vi "Traffic lights.vi"() -> ()   [LabVIEW 2012]
doc: "Use this template to build a standard state machine design pattern. Each state executes code and determines which state to transition to. Contrast this design pattern with the User Interface Event Handler pattern, in which code executes in response to user actions. Contrast this design pattern also with the Queued Message Handler pattern, in which each message handling code can queue zero or more new messages.\nNote: This template does not contain the most recent programming guidelines recommended by National Instruments. For a complete, project-based implementation of the Standard State Machine pattern, use the Create Project dialog box instead of this template."
uses:
  swiatla.ctl
  <vilib>/DAQmx/write.llb/DAQmx Write (Digital 1D Bool 1Chan 1Samp).vi
  <vilib>/DAQmx/create/channels.llb/DAQmx Create Channel (DO-Digital Output).vi
  <vilib>/DAQmx/miscellaneous.llb/DAQmx Fill In Error Info.vi
panel:
  in  "Numeric":dbl=20.0
  in  "pomaranczowe":bool
  in  "stop":bool
  in  "DAQmx Physical Channel":tag="Dev4/port0/line0:5"
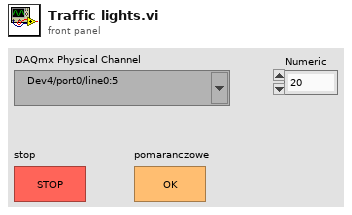
[diagram p1: front panel]
types:
  T1 = typedef "swiatla.ctl" = enum16{"Initialize", "Czerwone", "Czerwono-pomaranczowe", "Zielone", "Pomaranczowe", "Migajace_pomarancz", "Podw_czerw", "Powd_czerw_pomaran", "Mig_zgasz", "Stop"}
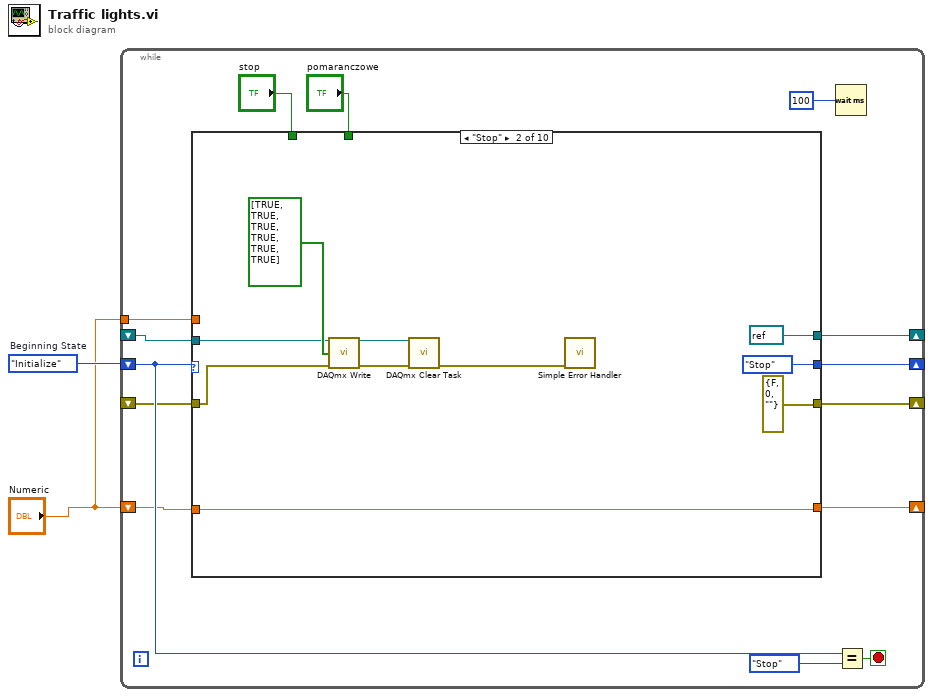
[diagram p0: block diagram]
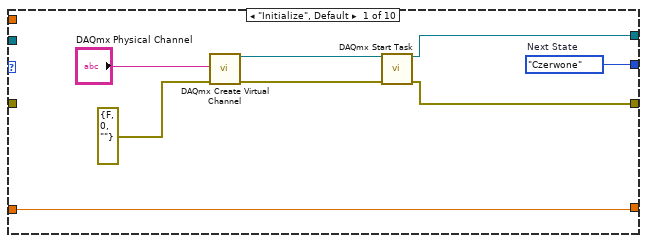
[diagram p2: hidden frame]
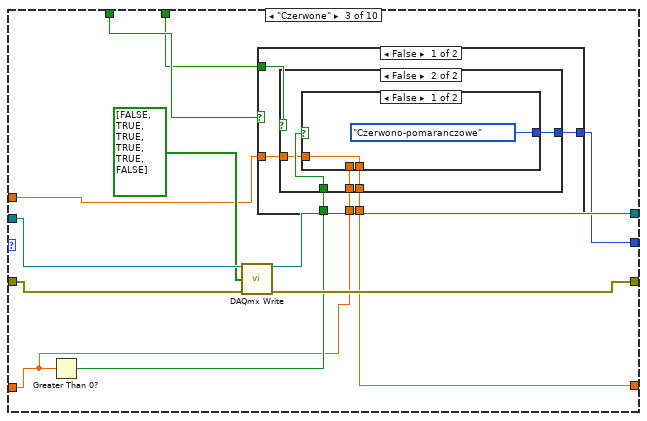
[diagram p3: hidden frame]
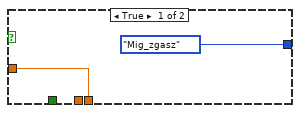
[diagram p4: hidden frame]
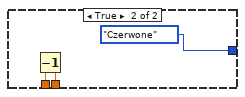
[diagram p5: hidden frame]
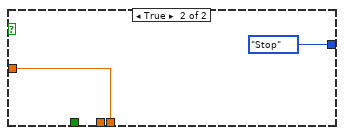
[diagram p6: hidden frame]
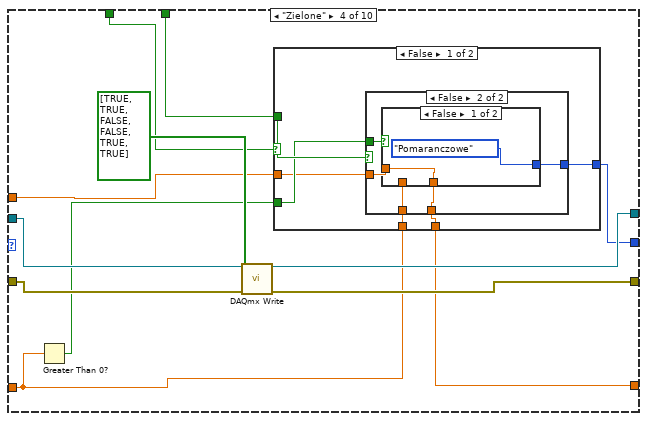
[diagram p7: hidden frame]
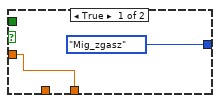
[diagram p8: hidden frame]
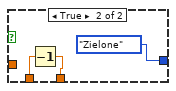
[diagram p9: hidden frame]
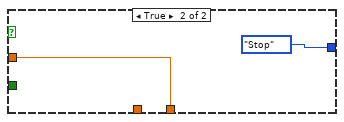
[diagram p10: hidden frame]
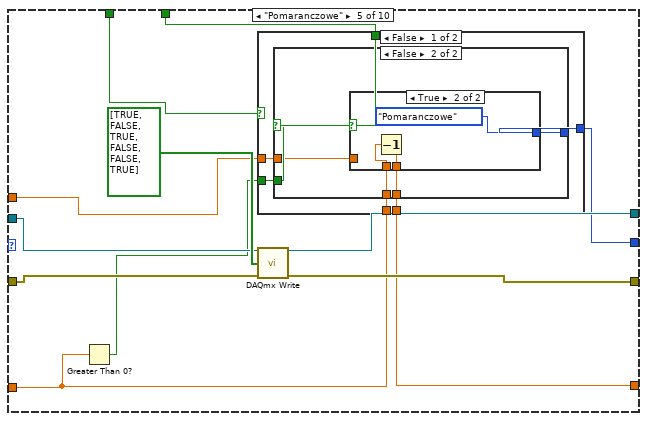
[diagram p11: hidden frame]
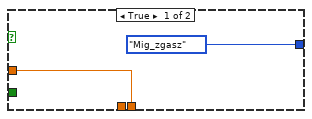
[diagram p12: hidden frame]
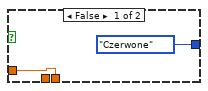
[diagram p13: hidden frame]
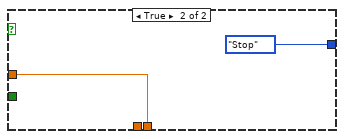
[diagram p14: hidden frame]
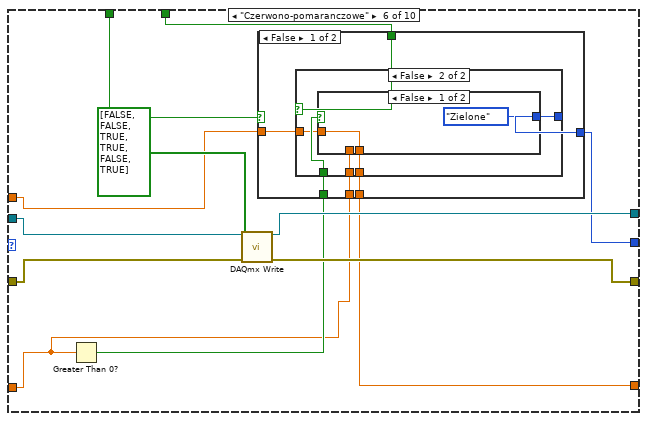
[diagram p15: hidden frame]
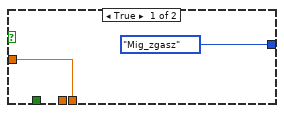
[diagram p16: hidden frame]
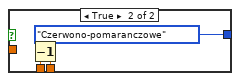
[diagram p17: hidden frame]
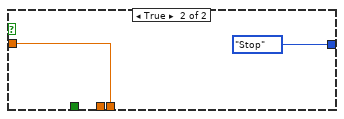
[diagram p18: hidden frame]
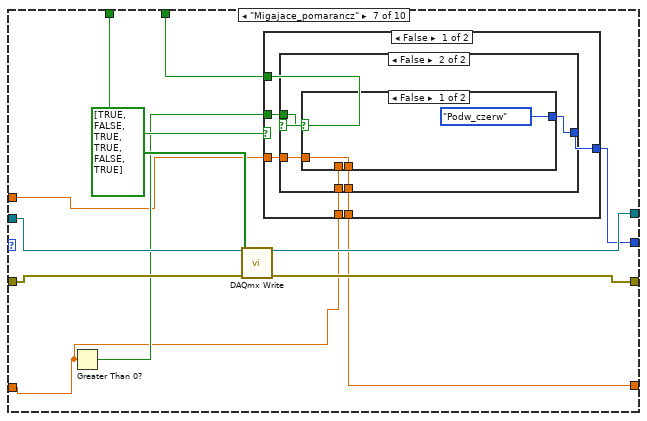
[diagram p19: hidden frame]
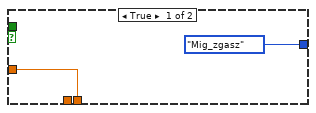
[diagram p20: hidden frame]
diagram:
  w2 = swiatla."Initialize"  # Beginning State
  n1 = while {
    shift-right: [w13] -> _
    shift-left: w2 -> [w14]
    shift-right: [w10] -> _
    shift-left: _ -> [w8]
    shift-right: [w11] -> _
    shift-left: _ -> [w9]
    shift-right: [w4] -> _
    shift-left: "Numeric" -> [w5]
    tunnel: "Numeric" -> [w3]
    stop <- w16 stop-if-true
    n2 = case shown="\"Stop\"" w14 {
      tunnel: [w24 swiatla."Stop" ("Next State") w40 w72 w104 w136 w168 w200 w232 w264] -> w13
      tunnel: [w20 refnum<k21> refnum ("task out") w43 w74 w109 w138 w170 w202 w234 w266] -> w11
      tunnel: [w19 errorcluster {"status"=FALSE, "code"=0, "source"=""} ("error out") w42 w75 w108 w139 w169 w201 w233 w265] -> w10
      tunnel: w9 -> [_ w29 w46 w77 w107 w141 w172 w204 w236 w268]
      tunnel: w8 -> [_ w28 w45 w76 w106 w140 w171 w203 w235 w267]
      tunnel: "stop" -> [_ _ w41 w73 w105 w137 w173 w205 w237 w269]
      tunnel: "pomaranczowe" -> [_ _ w39 w71 w103 w135 w167 w199 w231 w263]
      tunnel: w5 -> [w17 w25 w37 w69 w101 w133 w165 w197 w229 w261]
      tunnel: [w17 w25 w36 w68 w100 w132 w164 w196 w228 w260] -> w4
      tunnel: w3 -> [_ _ w35 w67 w99 w131 w163 w195 w227 w259]
      frame "Initialize", Default {
        w24 = swiatla."Czerwone"  # Next State
        n3 = call-poly <vilib>:"DAQmx Create Virtual Channel.vi"("lines"="DAQmx Physical Channel", "error in"=errorcluster {"status"=FALSE, "code"=0, "source"=""}) -> ("task out"=w22:refnum<k21>, "error out"=w21:errorcluster)  [unwired: 12 in]
        n4 = call <vilib>:"DAQmx Start Task.vi"("task/channels in"=w22, "error in"=w21) -> ("task out"=w20:refnum<k21>, "error out"=w19:errorcluster)  [unwired: 12 in]
      }
      frame "Stop" {
        n5 = call-poly <vilib>:"DAQmx Write.vi"("task/channels in"=w29, "data"=bool[] [TRUE, TRUE, TRUE, TRUE, TRUE, TRUE], "error in"=w28) -> ("task out"=w31:refnum<k21>, "error out"=w30:errorcluster)  [unwired: 10 in, 1 out]
        n6 = call <vilib>:"DAQmx Clear Task.vi"("task in"=w31, "error in"=w30) -> ("error out"=w33:errorcluster)  [unwired: 13 in]
        n7 = call <vilib>:"Simple Error Handler.vi"("error in (no error)"=w33) -> ()  [unwired: 4 in, 5 out]
      }
      frame "Czerwone" {
        n8 = Greater Than 0?(x=w37) -> (x > 0?=w38:bool)
        n9 = call-poly <vilib>:"DAQmx Write.vi"("task/channels in"=w46, "data"=bool[] [FALSE, TRUE, TRUE, TRUE, TRUE, FALSE], "error in"=w45) -> ("task out"=w43:refnum<k21>, "error out"=w42:errorcluster)  [unwired: 10 in, 1 out]
        n10 = case shown="False" w41 {
          tunnel: [w52 swiatla."Stop" ("Next State")] -> w40
          tunnel: w39 -> [w51 _]
          tunnel: w38 -> [w50 _]
          tunnel: w37 -> [w49 _]
          tunnel: [w48 w65] -> w36
          tunnel: w35 -> [w47 w65]
          frame False {
            n11 = case shown="False" w51 {
              tunnel: [swiatla."Mig_zgasz" ("Next State") w59] -> w52
              tunnel: w50 -> [_ w58]
              tunnel: w49 -> [_ w57]
              tunnel: [w53 w56] -> w48
              tunnel: w47 -> [w53 w55]
              frame True {
              }
              frame False {
                n12 = case shown="False" w58 {
                  tunnel: [swiatla."Czerwono-pomaranczowe" ("Next State") swiatla."Czerwone" ("Next State")] -> w59
                  tunnel: w57 -> [_ w63]
                  tunnel: [w60 w62] -> w56
                  tunnel: w55 -> [w60 _]
                  frame False {
                  }
                  frame True {
                    n13 = Decrement(x=w63) -> (x-1=w62:dbl)
                  }
                }
              }
            }
          }
          frame True {
          }
        }
      }
      frame "Zielone" {
        n14 = Greater Than 0?(x=w69) -> (x > 0?=w70:bool)
        n15 = call-poly <vilib>:"DAQmx Write.vi"("task/channels in"=w77, "data"=bool[] [TRUE, TRUE, FALSE, FALSE, TRUE, TRUE], "error in"=w76) -> ("task out"=w74:refnum<k21>, "error out"=w75:errorcluster)  [unwired: 10 in, 1 out]
        n16 = case shown="False" w73 {
          tunnel: [w84 swiatla."Stop" ("Next State")] -> w72
          tunnel: w71 -> [w83 _]
          tunnel: w70 -> [w82 _]
          tunnel: w69 -> [w81 _]
          tunnel: [w80 w97] -> w68
          tunnel: w67 -> [w79 w97]
          frame False {
            n17 = case shown="False" w83 {
              tunnel: [swiatla."Mig_zgasz" ("Next State") w91] -> w84
              tunnel: w82 -> [_ w90]
              tunnel: w81 -> [_ w89]
              tunnel: [w85 w88] -> w80
              tunnel: w79 -> [w85 w87]
              frame True {
              }
              frame False {
                n18 = case shown="False" w90 {
                  tunnel: [swiatla."Pomaranczowe" ("Next State") swiatla."Zielone" ("Next State")] -> w91
                  tunnel: w89 -> [_ w95]
                  tunnel: [w92 w94] -> w88
                  tunnel: w87 -> [w92 _]
                  frame False {
                  }
                  frame True {
                    n19 = Decrement(x=w95) -> (x-1=w94:dbl)
                  }
                }
              }
            }
          }
          frame True {
          }
        }
      }
      frame "Pomaranczowe" {
        n20 = Greater Than 0?(x=w101) -> (x > 0?=w102:bool)
        n21 = case shown="False" w105 {
          tunnel: [w116 swiatla."Stop" ("Next State")] -> w104
          tunnel: w103 -> [w115 _]
          tunnel: w102 -> [w114 _]
          tunnel: w101 -> [w113 _]
          tunnel: [w112 w129] -> w100
          tunnel: w99 -> [w111 w129]
          frame False {
            n22 = case shown="False" w115 {
              tunnel: [swiatla."Mig_zgasz" ("Next State") w123] -> w116
              tunnel: w114 -> [_ w122]
              tunnel: w113 -> [_ w121]
              tunnel: [w117 w120] -> w112
              tunnel: w111 -> [w117 w119]
              frame True {
              }
              frame False {
                n23 = case shown="True" w122 {
                  tunnel: [swiatla."Czerwone" ("Next State") swiatla."Pomaranczowe" ("Next State")] -> w123
                  tunnel: w121 -> [_ w127]
                  tunnel: [w124 w126] -> w120
                  tunnel: w119 -> [w124 _]
                  frame False {
                  }
                  frame True {
                    n24 = Decrement(x=w127) -> (x-1=w126:dbl)
                  }
                }
              }
            }
          }
          frame True {
          }
        }
        n25 = call-poly <vilib>:"DAQmx Write.vi"("task/channels in"=w107, "data"=bool[] [TRUE, FALSE, TRUE, FALSE, FALSE, TRUE], "error in"=w106) -> ("task out"=w109:refnum<k21>, "error out"=w108:errorcluster)  [unwired: 10 in, 1 out]
      }
      frame "Czerwono-pomaranczowe" {
        n26 = Greater Than 0?(x=w133) -> (x > 0?=w134:bool)
        n27 = call-poly <vilib>:"DAQmx Write.vi"("task/channels in"=w141, "data"=bool[] [FALSE, FALSE, TRUE, TRUE, FALSE, TRUE], "error in"=w140) -> ("task out"=w138:refnum<k21>, "error out"=w139:errorcluster)  [unwired: 10 in, 1 out]
        n28 = case shown="False" w137 {
          tunnel: [w148 swiatla."Stop" ("Next State")] -> w136
          tunnel: w135 -> [w147 _]
          tunnel: w134 -> [w146 _]
          tunnel: w133 -> [w145 _]
          tunnel: [w144 w161] -> w132
          tunnel: w131 -> [w143 w161]
          frame False {
            n29 = case shown="False" w147 {
              tunnel: [swiatla."Mig_zgasz" ("Next State") w155] -> w148
              tunnel: w146 -> [_ w154]
              tunnel: w145 -> [_ w153]
              tunnel: [w149 w152] -> w144
              tunnel: w143 -> [w149 w151]
              frame True {
              }
              frame False {
                n30 = case shown="False" w154 {
                  tunnel: [swiatla."Zielone" ("Next State") swiatla."Czerwono-pomaranczowe" ("Next State")] -> w155
                  tunnel: w153 -> [_ w159]
                  tunnel: [w156 w158] -> w152
                  tunnel: w151 -> [w156 _]
                  frame False {
                  }
                  frame True {
                    n31 = Decrement(x=w159) -> (x-1=w158:dbl)
                  }
                }
              }
            }
          }
          frame True {
          }
        }
      }
      frame "Migajace_pomarancz" {
        n32 = Greater Than 0?(x=w165) -> (x > 0?=w166:bool)
        n33 = call-poly <vilib>:"DAQmx Write.vi"("task/channels in"=w172, "data"=bool[] [TRUE, FALSE, TRUE, TRUE, FALSE, TRUE], "error in"=w171) -> ("task out"=w170:refnum<k21>, "error out"=w169:errorcluster)  [unwired: 10 in, 1 out]
        n34 = case shown="False" w173 {
          tunnel: [w180 swiatla."Stop" ("Next State")] -> w168
          tunnel: w167 -> [w179 _]
          tunnel: w166 -> [w178 _]
          tunnel: w165 -> [w177 _]
          tunnel: [w176 w193] -> w164
          tunnel: w163 -> [w175 w193]
          frame False {
            n35 = case shown="False" w179 {
              tunnel: [swiatla."Mig_zgasz" ("Next State") w187] -> w180
              tunnel: w178 -> [_ w186]
              tunnel: w177 -> [_ w185]
              tunnel: [w181 w184] -> w176
              tunnel: w175 -> [w181 w183]
              frame True {
              }
              frame False {
                n36 = case shown="False" w186 {
                  tunnel: [swiatla."Podw_czerw" ("Next State") swiatla."Migajace_pomarancz" ("Next State")] -> w187
                  tunnel: w185 -> [_ w191]
                  tunnel: [w188 w190] -> w184
                  tunnel: w183 -> [w188 _]
                  frame False {
                  }
                  frame True {
                    n37 = Decrement(x=w191) -> (x-1=w190:dbl)
                  }
                }
              }
            }
          }
          frame True {
          }
        }
      }
      frame "Mig_zgasz" {
        n38 = Greater Than 0?(x=w197) -> (x > 0?=w198:bool)
        n39 = call-poly <vilib>:"DAQmx Write.vi"("task/channels in"=w204, "data"=bool[] [TRUE, TRUE, TRUE, TRUE, TRUE, TRUE], "error in"=w203) -> ("task out"=w202:refnum<k21>, "error out"=w201:errorcluster)  [unwired: 10 in, 1 out]
        n40 = case shown="False" w205 {
          tunnel: [w212 swiatla."Stop" ("Next State")] -> w200
          tunnel: w199 -> [w211 _]
          tunnel: w198 -> [w210 _]
          tunnel: w197 -> [w209 _]
          tunnel: [w208 w225] -> w196
          tunnel: w195 -> [w207 w225]
          frame False {
            n41 = case shown="False" w211 {
              tunnel: [swiatla."Migajace_pomarancz" ("Next State") w219] -> w212
              tunnel: w210 -> [_ w218]
              tunnel: w209 -> [_ w217]
              tunnel: [w213 w216] -> w208
              tunnel: w207 -> [w213 w215]
              frame True {
              }
              frame False {
                n42 = case shown="False" w218 {
                  tunnel: [swiatla."Podw_czerw" ("Next State") swiatla."Mig_zgasz" ("Next State")] -> w219
                  tunnel: w217 -> [_ w223]
                  tunnel: [w220 w222] -> w216
                  tunnel: w215 -> [w220 _]
                  frame False {
                  }
                  frame True {
                    n43 = Decrement(x=w223) -> (x-1=w222:dbl)
                  }
                }
              }
            }
          }
          frame True {
          }
        }
      }
      frame "Podw_czerw" {
        n44 = Greater Than 0?(x=w229) -> (x > 0?=w230:bool)
        n45 = call-poly <vilib>:"DAQmx Write.vi"("task/channels in"=w236, "data"=bool[] [FALSE, TRUE, TRUE, FALSE, TRUE, TRUE], "error in"=w235) -> ("task out"=w234:refnum<k21>, "error out"=w233:errorcluster)  [unwired: 10 in, 1 out]
        n46 = case shown="False" w237 {
          tunnel: [w244 swiatla."Stop" ("Next State")] -> w232
          tunnel: w231 -> [w243 _]
          tunnel: w230 -> [w242 _]
          tunnel: w229 -> [w241 _]
          tunnel: [w240 w257] -> w228
          tunnel: w227 -> [w239 w257]
          frame False {
            n47 = case shown="False" w243 {
              tunnel: [swiatla."Mig_zgasz" ("Next State") w251] -> w244
              tunnel: w242 -> [_ w250]
              tunnel: w241 -> [_ w249]
              tunnel: [w245 w248] -> w240
              tunnel: w239 -> [w245 w247]
              frame True {
              }
              frame False {
                n48 = case shown="False" w250 {
                  tunnel: [swiatla."Powd_czerw_pomaran" ("Next State") swiatla."Podw_czerw" ("Next State")] -> w251
                  tunnel: w249 -> [_ w255]
                  tunnel: [w252 w254] -> w248
                  tunnel: w247 -> [w252 _]
                  frame False {
                  }
                  frame True {
                    n49 = Decrement(x=w255) -> (x-1=w254:dbl)
                  }
                }
              }
            }
          }
          frame True {
          }
        }
      }
      frame "Powd_czerw_pomaran" {
        n50 = Greater Than 0?(x=w261) -> (x > 0?=w262:bool)
        n51 = call-poly <vilib>:"DAQmx Write.vi"("task/channels in"=w268, "data"=bool[] [FALSE, FALSE, TRUE, FALSE, TRUE, TRUE], "error in"=w267) -> ("task out"=w266:refnum<k21>, "error out"=w265:errorcluster)  [unwired: 10 in, 1 out]
        n52 = case shown="False" w269 {
          tunnel: [w276 swiatla."Stop" ("Next State")] -> w264
          tunnel: w263 -> [w275 _]
          tunnel: w262 -> [w274 _]
          tunnel: w261 -> [w273 _]
          tunnel: [w272 w289] -> w260
          tunnel: w259 -> [w271 w289]
          frame False {
            n53 = case shown="False" w275 {
              tunnel: [swiatla."Mig_zgasz" ("Next State") w283] -> w276
              tunnel: w274 -> [_ w282]
              tunnel: w273 -> [_ w281]
              tunnel: [w277 w280] -> w272
              tunnel: w271 -> [w277 w279]
              frame True {
              }
              frame False {
                n54 = case shown="False" w282 {
                  tunnel: [swiatla."Zielone" ("Next State") swiatla."Powd_czerw_pomaran" ("Next State")] -> w283
                  tunnel: w281 -> [_ w287]
                  tunnel: [w284 w286] -> w280
                  tunnel: w279 -> [w284 _]
                  frame False {
                  }
                  frame True {
                    n55 = Decrement(x=w287) -> (x-1=w286:dbl)
                  }
                }
              }
            }
          }
          frame True {
          }
        }
      }
    }
    n56 = Wait (ms)(milliseconds to wait=u32 100) -> ()  [unwired: 1 out]
    n57 = Equal?(x=w14, y=swiatla."Stop" ("States")) -> (x = y?=w16:bool)
  }
